vi "set_overlay.vi"(4 "error in (no error)":errorcluster, 5 "Value":T7={"overlay array"=[], "overlay name"="", "color (red)"=16711680, "overlay size"=0, "overlay type"=enum."crosshair"} {"overlay size" min=1}, 6 "Container State":T10, 7 "Display State In":T1 {"array of overlays"."overlay size" min=1}) -> (0 "error out":errorcluster, 3 "Display State Out":T1 {"array of overlays"."overlay size" min=1})   [LabVIEW 2010, in "XImage.xctl"]
uses:
  XImage.xctl
  <vilib>/_xctls/Container State.ctl
  overlays_cluster.ctl
  state.ctl
  classes/SpaceVector/SpaceVector/SpaceVector.lvclass
  classes/PointCollection/PointCollection/PointCollection.lvclass
  ROI_frames_cluster.ctl
  control_refs_cluster.ctl
  calibration_cluster.ctl
  enumerations/unit.ctl
  xpath_cluster.ctl
  ROI_mode_enum.ctl
  last_action_enum.ctl
  <vilib>/_xctls/XControlSupport.lvlib
  classes/Image/Image/Image.lvclass
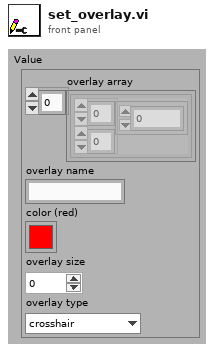
[diagram p1: front panel]
types:
  T1 = typedef "XImage.xctl/state.ctl" = cluster{"current frame index":i32, "number of images":i32, "ROI (frames)":T2, "control refs":T3, "calibration":T4, "xpaths":T6, "offset":refnum<class "SpaceVector.lvclass">, "XML description":string, "number of ROIs":dbl, "ROI Tool Buttons Visible":cluster{"Zoom Tool":bool, "Selection Tool":bool, "Pan Tool":bool, "Point Tool":bool, "Line Tool":bool, "Rectangle Tool":bool, "Rotated Rectangle Tool":bool, "Polyline Tool":bool, "Polygon Tool":bool, "Freehand Tool":bool, "Closed Freehand Tool":bool, "Ellipse Tool":bool, "Annulus Tool":bool}, "ROI color":u32, "enable ROI numbering?":bool, "selected path to save ROIs":path, "starting path":path, "array of overlays":T7[], "pointCollection":refnum<class "PointCollection.lvclass">, "ROImode":T8, "selected point ID":dbl, "point radius":i32, "point colours":u32[], "PlotAreaSize":cluster{"Width":u32, "Height":u32}, "last action":T9}
  T2 = typedef "XImage.xctl/ROI_frames_cluster.ctl" = cluster{"ROI":cluster{"Global Rectangle":i32[], "Contours":cluster{"Contour Type":u32, "ROI Type":u32, "Points":i32[]}[]}[]}
  T3 = typedef "XImage.xctl/control_refs_cluster.ctl" = cluster{"frame":refnum<vi>, "image":refnum<vi>, "saveROIsButton":refnum<vi>, "loadImageSwitch":refnum<vi>, "loadROIsSwitch":refnum<vi>, "saveROIsSwitch":refnum<vi>, "loadImagePath":refnum<vi>, "loadROIPath":refnum<vi>, "redraw":refnum<vi>}
  T4 = typedef "XImage.xctl/calibration_cluster.ctl" = cluster{"x":dbl, "y":dbl, "x unit":T5, "y unit":T5}
  T5 = typedef "Image.lvclass/unit.ctl" = enum16{"um", "s"}
  T6 = typedef "XImage.xctl/xpath_cluster.ctl" = cluster{"x offset":string, "y offset":string, "z offset":string}
  T7 = typedef "XImage.xctl/overlays_cluster.ctl" = cluster{"overlay array":cluster{i32[][]}[], "overlay name":string, "color (red)":u32, "overlay size":i32, "overlay type":enum16{"crosshair", "circle"}}
  T8 = typedef "XImage.xctl/ROI_mode_enum.ctl" = enum16{"none", "IMAQROIs", "PointCollection"}
  T9 = typedef "XImage.xctl/last_action_enum.ctl" = enum16{"not specified", "image loaded", "frame changed", "ROIs changed"}
  T10 = typedef "XControlSupport.lvlib/Container State.ctl" = cluster{"Indicator?":bool, "Run Mode?":bool, " Refnum":refnum<vi>}
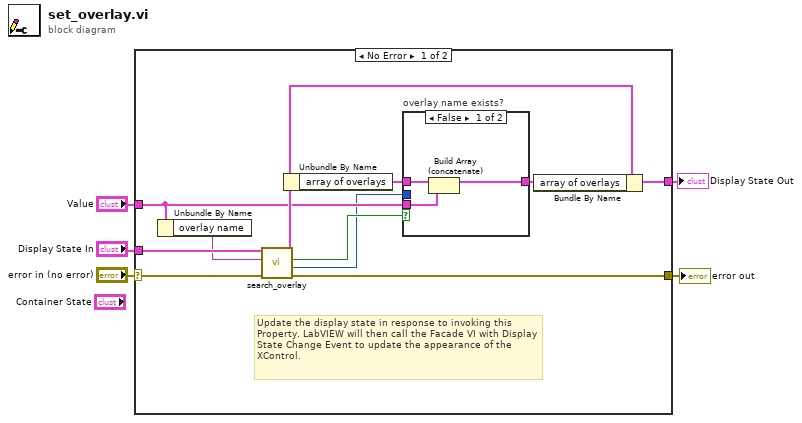
[diagram p0: block diagram]
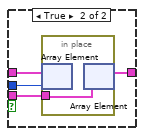
[diagram p2: hidden frame]
diagram:
  n1 = case shown="No Error" "error in (no error)" {
    selector: "error in (no error)" -> [w13 w26]
    tunnel: [w6 w26] -> w4
    tunnel: [w12 w25] -> w5
    tunnel: "Display State In" -> [w16 w25]
    tunnel: "Value" -> [w9 _]
    frame No Error {
      # "Update the display state in response to invoking this Property. LabVIEW will then call the Facade VI with Display State Change Event to update the appearance of the XControl."
      n2 = Unbundle By Name(w9) -> ("overlay name"=w8:string)
      n3 = call "search_overlay.vi"("error in (no error)"=w13, "overlay name"=w8, "Display State In"=w16) -> ("error out"=w6:errorcluster, "index"=w7:i32, "found?"=w14:bool, "Display State Out"=w15:T1)  [unwired: 5 in]
      n4 = Unbundle By Name(w15) -> ("array of overlays"=w11:T7[])
      n5 = case "overlay name exists?" shown="False" w14 {
        tunnel: w11 -> [w18 w23]
        tunnel: w7 -> [_ w22]
        tunnel: [w19 w21] -> w10
        tunnel: w9 -> [w17 w20]
        frame False {
          n6 = Build Array (concatenate)(w18, w17) -> (w19:T7[])
        }
        frame True {
          n7 = in-place {
            in-place-border: w20 -> [w24]
            n8 = in-place-array #1(w23, w22) -> ()  [unwired: 1 out]
            n9 = in-place-array #1(w24) -> (w21:T7[])  [unwired: 1 out]
          }
        }
      }
      n10 = Bundle By Name(cluster=w15, "array of overlays"=w10) -> (w12:T1)
    }
    frame Error {
    }
  }
  "error out" <- w4
  "Display State Out" <- w5
